vi "HMI Pop Up Num KP.vi"(4 "Password Display (F)":bool, 6 "Max Length (50)":i32=50, 9 "Text":string, 10 "String In":string, 11 "Message In":string) -> (1 "Canceled":bool, 2 "String Out":string)   [LabVIEW 2015, in "Touch_keyboard.lvlib"]
doc: "Name: Pop Up Keypad\nAuthor:Georges Janveau, Columbia Forest Products\n\n\nDESCRIPTION\nSimulates a numeric keypad intended to be used on a touchscreen PC. The input control can be set for standard or password display.\n\nINPUTS\nMessage In - Optional message displayed in the title bar.\nString In - Sets the initial value of the edit box.\nPassword Display (F) - Sets standard or password display.\nMax Length (50) - Sets the maximum length allowed in the edit box.\n\nOUTPUTS\nString Out - Result (will contain String In if the user cancels).\nCanceled - True if the user cancels.\n\n----------------------------------------------------------------------------------------------------------------"
uses:
  Touch_keyboard.lvlib
  Driver Commands.ctl
panel:
  in  ".":bool
  in  "0":bool
  in  "3":bool
  in  "2":bool
  in  "1":bool
  in  "6":bool
  in  "5":bool
  in  "4":bool
  in  "9":bool
  in  "8":bool
  in  "7":bool
  in  "Right":bool
  in  "Left":bool
  in  "Ok":bool
  in  "Cancel":bool
  in  "Backspace":bool
  # "Inputs"
  # "Outputs"
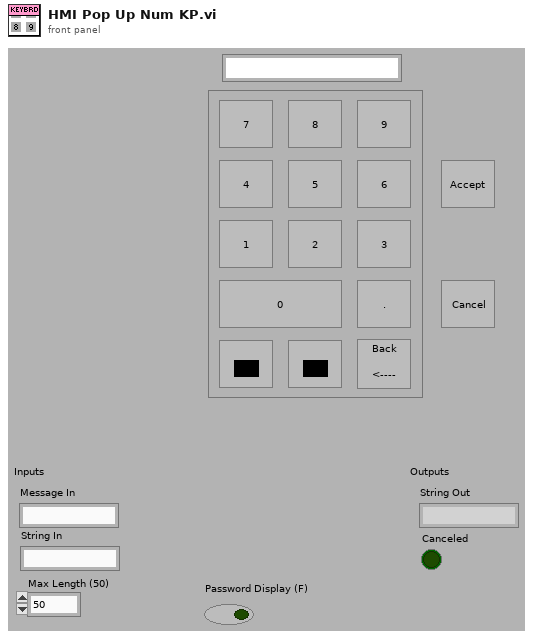
[diagram p1: front panel]
types:
  T1 = typedef "Touch_keyboard.lvlib/Driver Commands.ctl" = enum16{"No Command", "Initialize", "Add Character", "Replace Charcter", "Delete Character", "Move Left", "Move Right", "Update Edit Position"}
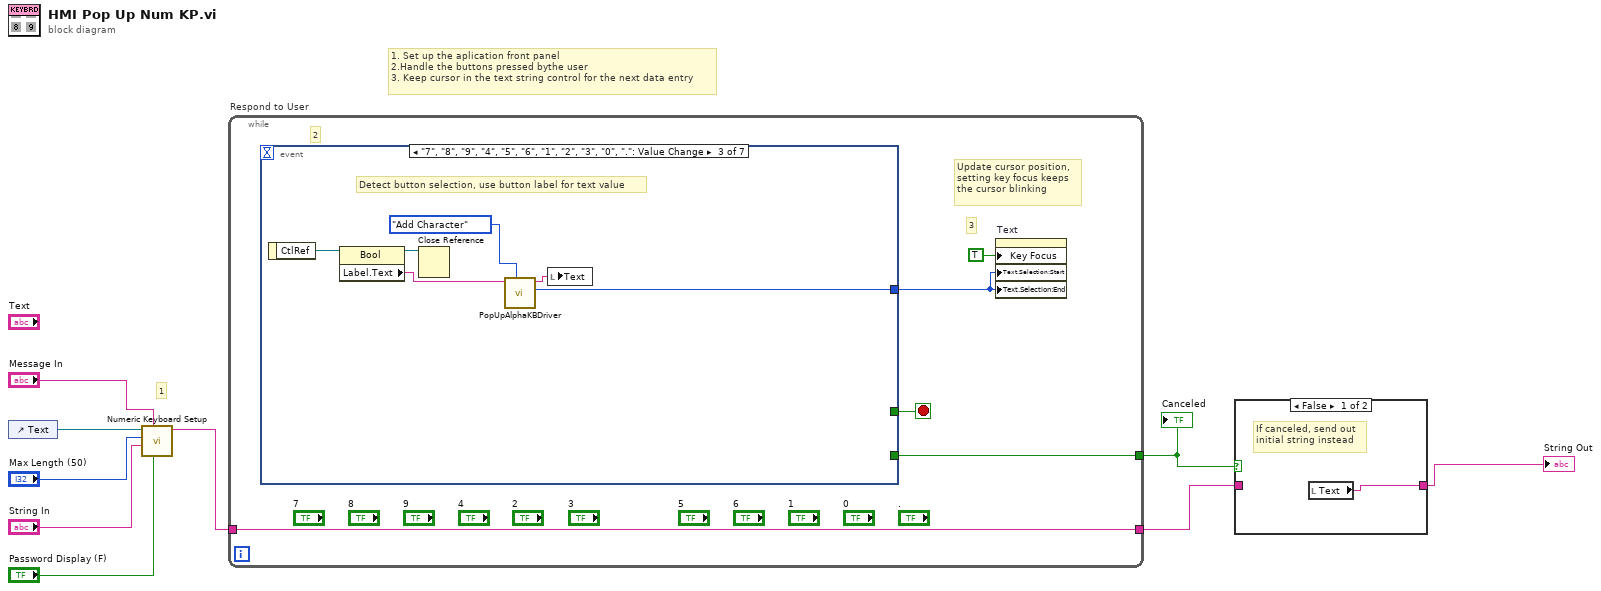
[diagram p0: block diagram]
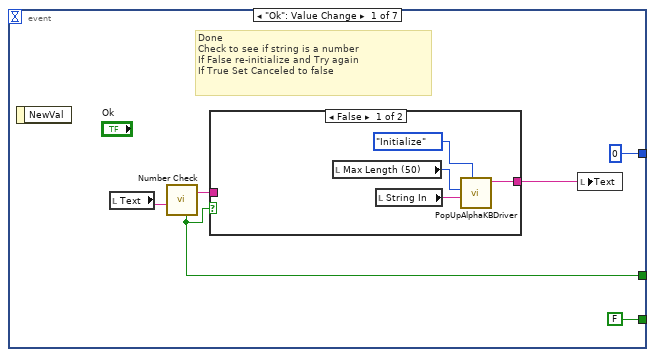
[diagram p3: hidden frame]
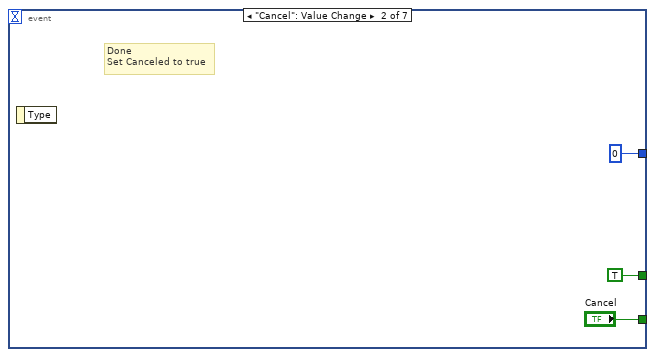
[diagram p5: hidden frame]
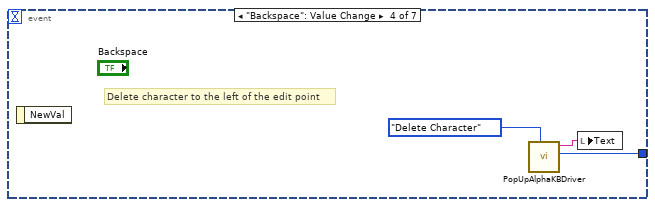
[diagram p6: hidden frame]
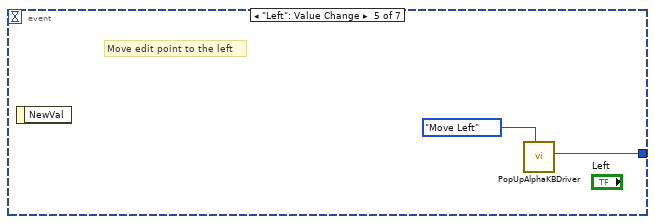
[diagram p7: hidden frame]
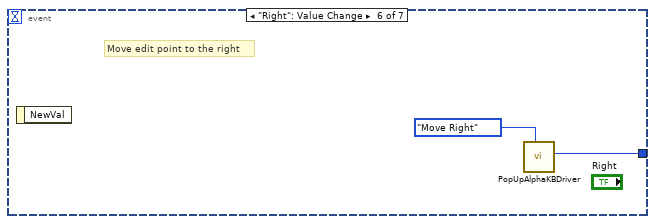
[diagram p8: hidden frame]
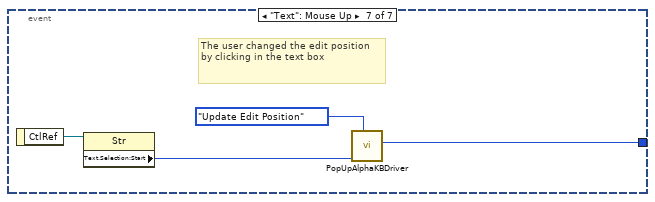
[diagram p9: hidden frame]
diagram:
  # "1. Set up the aplication front panel\n2.Handle the buttons pressed bythe user\n3. Keep cursor in the text string control for the next data entry"
  # "1"
  n1 = control-ref of="Text"() -> (w3:refnum<vi>)
  n2 = call "Numeric Keyboard Setup.vi"("Password Display (F)"="Password Display (F)", "Message In"="Message In", "String In"="String In", "Max Length (50)"="Max Length (50)", "String in"=w3) -> ("String Out"=w9:string)  [unwired: 5 in, 1 out]
  n3 = while "Respond to User" {
    tunnel: w9 -> [w11]
    tunnel: [w12] -> w1
    tunnel: [w11] -> w8
    stop <- w14 stop-if-true
    # "3"
    # "Update cursor position,\nsetting key focus keeps\nthe cursor blinking"
    # "2"
    n4 = event shown="[2] \"7\", \"8\", \"9\", \"4\", \"5\", \"6\", \"1\", \"2\", \"3\", \"0\", \".\": Value Change" {
      selector: _ -> [_ _ _ _ _ _ _]
      dyn-events: _ -> [_ _ _ _ _ _ _]
      timeout: _ -> [_ _ _ _ _ _ _]
      tunnel: [w15 TRUE _ _ _ _ _] -> w14
      tunnel: [0 ("Edit Position") 0 ("Edit Position") w32 w36 w39 w40 w42] -> w13
      tunnel: [FALSE ("Cancel") "Cancel" _ _ _ _ _] -> w12
      event "Ok": Value Change {
        # "Done\nCheck to see if string is a number\nIf False re-initialize and Try again\nIf True Set Canceled to false"
        n5 = event-data() -> ()  [unwired: 1 in, 1 out]
        n6 = local read "Text"() -> (w16:string)
        n7 = call "Number Check.vi"("string in"=w16) -> ("Number?"=w15:bool, "String out"=w17:string)  [unwired: 9 in]
        n8 = case shown="False" w15 {
          tunnel: w17 -> [_ w25]
          tunnel: [w21 w25] -> w18
          frame False {
            n9 = local read "Max Length (50)"() -> (w23:i32)
            n10 = local read "String In"() -> (w22:string)
            n11 = call "PopUpAlphaKBDriver.vi"("Driver Commands"=Driver_Commands."Initialize", "Initial String"=w22, "Max Length (70)"=w23) -> ("String Out"=w21:string)  [unwired: 7 in, 1 out]
          }
          frame True {
          }
        }
        n12 = local write "Text"(w18) -> ()
      }
      event "Cancel": Value Change {
        # "Done\nSet Canceled to true"
        n13 = event-data() -> ()  [unwired: 1 in, 1 out]
      }
      event "7", "8", "9", "4", "5", "6", "1", "2", "3", "0", ".": Value Change {
        # "Detect button selection, use button label for text value"
        n14 = event-data() -> ("CtlRef"=w34:refnum<vi>)  [unwired: 1 in]
        n15 = property class="Bool"(reference=w34) -> (reference out=w33:refnum<vi>, "Label.Text"=w29:string)  [unwired: 1 in, 1 out]
        n16 = Close Reference(reference=w33) -> ()  [unwired: 1 in, 1 out]
        n17 = call "PopUpAlphaKBDriver.vi"("Driver Commands"=Driver_Commands."Add Character", "Character"=w29) -> ("Edit Position"=w32:i32, "String Out"=w31:string)  [unwired: 8 in]
        n18 = local write "Text"(w31) -> ()
      }
      event "Backspace": Value Change {
        # "Delete character to the left of the edit point"
        n19 = event-data() -> ()  [unwired: 1 in, 1 out]
        n20 = call "PopUpAlphaKBDriver.vi"("Driver Commands"=Driver_Commands."Delete Character") -> ("Edit Position"=w36:i32, "String Out"=w35:string)  [unwired: 9 in]
        n21 = local write "Text"(w35) -> ()
      }
      event "Left": Value Change {
        # "Move edit point to the left"
        n22 = event-data() -> ()  [unwired: 1 in, 1 out]
        n23 = call "PopUpAlphaKBDriver.vi"("Driver Commands"=Driver_Commands."Move Left") -> ("Edit Position"=w39:i32)  [unwired: 9 in, 1 out]
      }
      event "Right": Value Change {
        # "Move edit point to the right"
        n24 = event-data() -> ()  [unwired: 1 in, 1 out]
        n25 = call "PopUpAlphaKBDriver.vi"("Driver Commands"=Driver_Commands."Move Right") -> ("Edit Position"=w40:i32)  [unwired: 9 in, 1 out]
      }
      event "Text": Mouse Up {
        # "The user changed the edit position\nby clicking in the text box"
        n26 = event-data() -> ("CtlRef"=w45:refnum<vi>)  [unwired: 1 in]
        n27 = property class="Str"(reference=w45) -> ("Text.Selection:Start"=w44:u32)  [unwired: 1 in, 2 out]
        n28 = call "PopUpAlphaKBDriver.vi"("Driver Commands"=Driver_Commands."Update Edit Position", "New Edit Position"=w44) -> ("Edit Position"=w42:i32)  [unwired: 8 in, 1 out]
      }
    }
    n29 = property on="Text" class="Str"("Key Focus"=TRUE, "Text.Selection:Start"=w13, "Text.Selection:End"=w13) -> ()  [unwired: 2 in, 2 out]
  }
  "Canceled" <- w1
  n30 = case shown="False" w1 {
    tunnel: w8 -> [_ w47]
    tunnel: [w46 w47] -> w2
    frame False {
      # "If canceled, send out\ninitial string instead"
      n31 = local read "Text"() -> (w46:string)
    }
    frame True {
    }
  }
  "String Out" <- w2
